vi "Elevator Control Loop.vi"() -> ()   [LabVIEW 2017]
uses:
  <vilib>/Rock Robotics/WPI/MotorControl/WPI_MotorControlDeviceRef.ctl
  <vilib>/Rock Robotics/WPI/MotorControl/WPI_MotorControlType.ctl
  <vilib>/Rock Robotics/SystemInterfaces/DIO/FPGA_DIOPWMChannel.ctl
  <vilib>/Rock Robotics/WPI/PWM/WPI_PWMDeadband.ctl
  <vilib>/Rock Robotics/SystemInterfaces/DIO/FPGA_DIOChannel.ctl
  <vilib>/Rock Robotics/WPI/Encoder/WPI_EncoderDevRef.ctl
  <vilib>/Rock Robotics/SystemInterfaces/Encoder/FPGA_EncoderIdx.ctl
  <vilib>/Rock Robotics/SystemInterfaces/Counter/FPGA_CounterCtrSystemIndex.ctl
  <vilib>/Rock Robotics/WPI/Encoder/WPI_EncoderType.ctl
  Typedef/Controller Message.ctl
  <vilib>/Platform/TimedLoop/XDataNode/timing_clust.ctl
  <vilib>/Platform/TimedLoop/XDataNode/nitl_modes.ctl
  <vilib>/Platform/TimedLoop/XDataNode/wakeup.ctl
  Typedef/FGVAction.ctl
  <vilib>/addons/control/pid/pid.llb/PID Advanced (DBL).vi
  SimulatorVIs/Simulation Input Global.vi
  <vilib>/Platform/TimedLoop/XDataNode/XDataNode.xnode
  <vilib>/Platform/TimedLoop/XDataNode/XDNodeRunTimeDep.lvlib
  <vilib>/addons/control/pid/NI_PID_pid.lvlib
panel:
  in  "min speed":dbl=0.1 format="%#_13g"
  in  "gravity":dbl=0.02 format="%#_13g"
  in  "PIDF gains":cluster{"Kp":dbl, "Ki":dbl, "Kd":dbl, "Kf":dbl}={"Kp"=0.01, "Ki"=0.0, "Kd"=0.06, "Kf"=0.0} {"Kf" format="%.3f"; "Kd" format="%.3f"; "Ki" format="%.3f"; "Kp" format="%.3f"}
  out "Plant Input":dbl(graph)=0.12000000000000001
  in  "output range":cluster{"output high":dbl, "output low":dbl}={"output high"=1.0, "output low"=-1.0} {"output low" format="%.2f"; "output high" format="%.2f"}
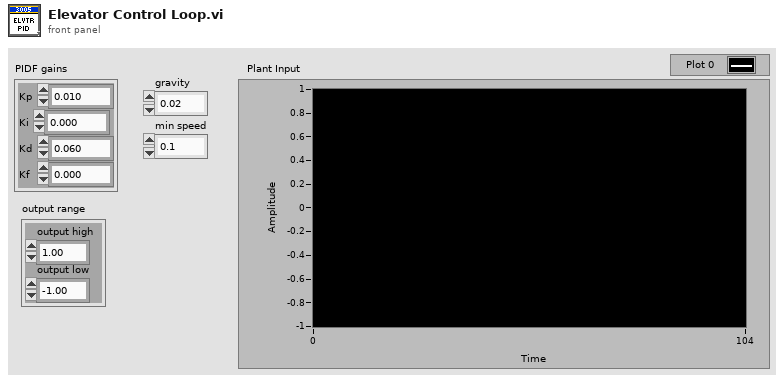
[diagram p1: front panel]
types:
  T1 = typedef "Controller Message.ctl" = cluster{"Setpoint":dbl, "Manual":bool}
  T2 = typedef "WPI_MotorControlDeviceRef.ctl" = cluster{"DeviceStatus":errorcluster, "Type":T3, "PWM":cluster{"PWM Channel":T4, "DeadBand":T5}, "CAN":cluster{"Device Number":u8, "SetOutput VI Ref":variant, "GetOutput VI Ref":variant, "Enable VI Ref":variant, "Disable VI Ref":variant, "Data":variant}, "Invert":bool, "DIO PWM":cluster{"PWM \"Enable\" Channel":T4, "DIOChannel":T6, "PWM Rate":dbl}}
  T3 = typedef "WPI_MotorControlType.ctl" = enum16{"PWM", "CAN", "DIO PWM"}
  T4 = typedef "FPGA_DIOPWMChannel.ctl" = enum8{"PWM 0", "PWM 1", "PWM 2", "PWM 3", "PWM 4", "PWM 5", "PWM 6", "PWM 7", "PWM 8", "PWM 9", "PWM MXP 0", "PWM MXP 1", "PWM MXP 2", "PWM MXP 3", "PWM MXP 4", "PWM MXP 5", "PWM MXP 6", "PWM MXP 7", "PWM MXP 8", "PWM MXP 9", "Invalid"}
  T5 = typedef "WPI_PWMDeadband.ctl" = cluster{"Name":string, "maxPositivePwm":i32, "minPositivePwm":i32, "centerPwm":i32, "maxNegativePwm":i32, "minNegativePwm":i32, "angularRange":u16}
  T6 = typedef "FPGA_DIOChannel.ctl" = enum8{"DIO 0", "DIO 1", "DIO 2", "DIO 3", "DIO 4", "DIO 5", "DIO 6", "DIO 7", "DIO 8", "DIO 9", "DIO MXP 0", "DIO MXP 1", "DIO MXP 2", "DIO MXP 3", "DIO MXP 4", "DIO MXP 5", "DIO MXP 6", "DIO MXP 7", "DIO MXP 8", "DIO MXP 9", "DIO MXP 10", "DIO MXP 11", "DIO MXP 12", "DIO MXP 13", "DIO MXP 14", "DIO MXP 15", "SPI Port CS1", "SPI Port CS2", "SPI Port CS3", "SPI Port MISO", "SPI Port MOSI", "Invalid"}
  T7 = typedef "WPI_EncoderDevRef.ctl" = cluster{"DevStatus":errorcluster, "EncoderIndex":T8, "CounterIndex":T9, "DistancePerCount":dbl, "Decoding Type":T10}
  T8 = typedef "FPGA_EncoderIdx.ctl" = enum8{"Enc 0", "Enc 1", "Enc 2", "Enc 3", "Enc 4", "Enc 5", "Enc 6", "Enc 7", "Invalid"}
  T9 = typedef "FPGA_CounterCtrSystemIndex.ctl" = enum8{"Ctr 0", "Ctr 1", "Ctr 2", "Ctr 3", "Ctr 4", "Ctr 5", "Ctr 6", "Ctr 7", "Invalid"}
  T10 = typedef "WPI_EncoderType.ctl" = enum16{"1x", "2x", "4x"}
  T11 = cluster{"Setpoint":dbl, "Output":dbl, "DriveMotor":T2, "Encoder":T7, "notifier":refnum<notifier>, "Manual?":bool}
  T12 = typedef "XDNodeRunTimeDep.lvlib/timing_clust.ctl" = cluster{"Expected End [f-1]":u64, "Actual End [f-1]":u64, "Finished Late? [f-1]":bool, "Expected End [i-1]":u64, "Actual End [i-1]":u64, "Finished Late? [i-1]":bool, "Expected Start [i]":u64, "Actual Start [i]":u64, "Expected Start [f]":u64, "Actual Start [f]":u64, "Source Name":string, "Structure Name":string, "Period":i64, "Deadline":i64, "Offset":i64, "Start":i64, "Priority":i32, "Timeout":i32, "Mode":T13, "Wakeup Reason":T14, "Error":errorcluster, "Source Type":string, "Secondary Source Type":string, "Global End Time":u64, "Global Start Time":u64, "Frame Duration":u64, "Iteration Duration":u64, "Assigned CPU":i32, "I/O Scan Engine Mode":u32}
  T13 = typedef "XDNodeRunTimeDep.lvlib/nitl_modes.ctl" = enum32{"No Change", "Process missed periods, maintain original phase", "Discard missed periods, maintain original phase", "Process missed periods, ignore original phase", "Discard missed periods, ignore original phase"}
  T14 = typedef "XDNodeRunTimeDep.lvlib/wakeup.ctl" = enum32{"Normal", "Aborted", "Asynchronous wakeup", "Timing source error", "Timed loop error", "Timeout"}
  T15 = typedef "FGVAction.ctl" = enum16{"get", "set"}
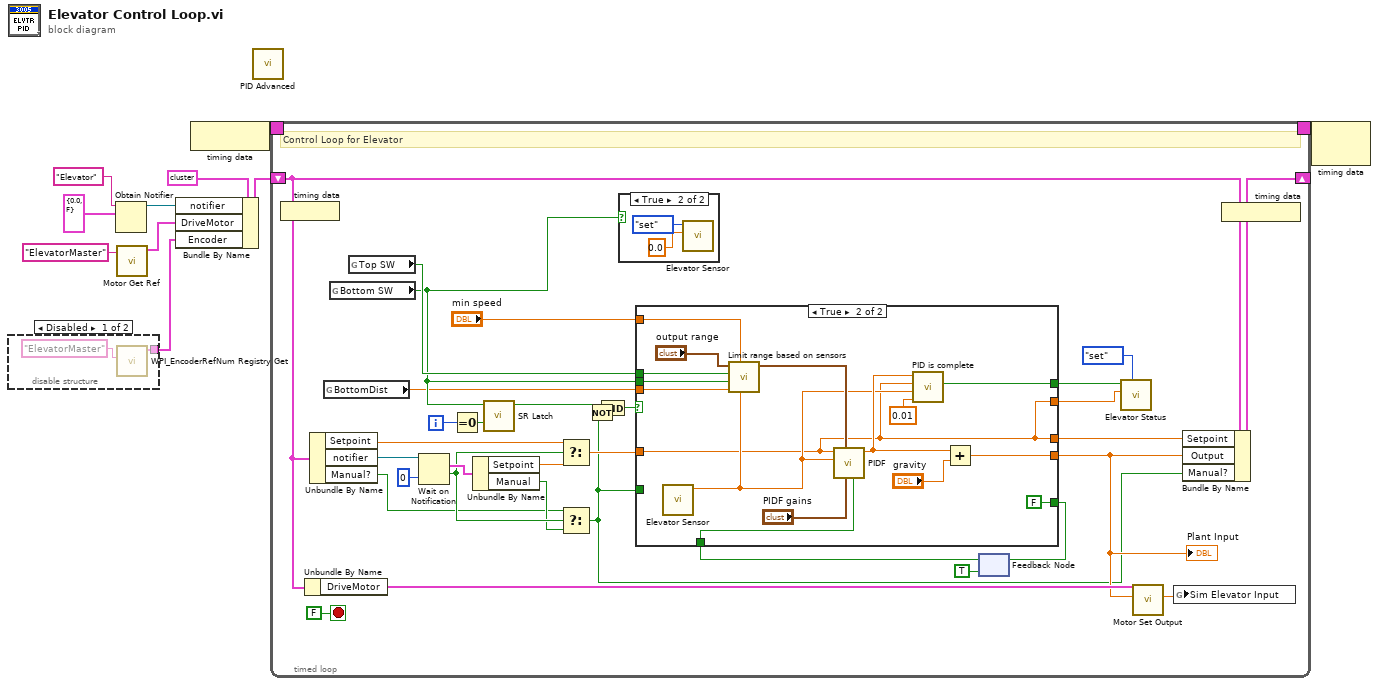
[diagram p0: block diagram]
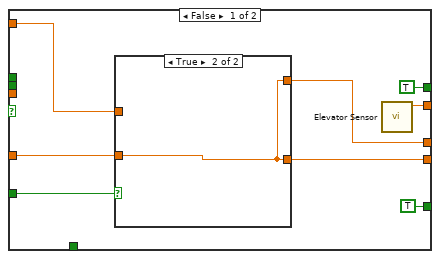
[diagram p3: hidden frame]
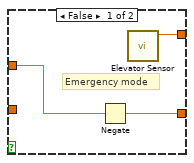
[diagram p4: hidden frame]
diagram:
  n1 = disable-structure shown="Disabled" {
    disable-tunnel: [w11 _] -> w4
    frame Disabled {
      n2 = call <vilib>:"WPI_EncoderRefNum Registry Get.vi"("refnum name"="ElevatorMaster") -> ("EncoderDevRef"=w11:T7)  [unwired: 9 in, 1 out]
    }
    frame Enabled {
    }
  }
  n3 = Obtain Notifier(name (unnamed)="Elevator", notification data type=T1 {"Setpoint"=0.0, "Manual"=FALSE}) -> (notifier out=w8:refnum<notifier>)  [unwired: 2 in, 2 out]
  n4 = call "Motor Get Ref.vi"("refnum name"="ElevatorMaster") -> ("MotorControlDevRef"=w6:T2)  [unwired: 10 in]
  n5 = Bundle By Name(cluster=T11 {"Setpoint"=0.0, "Output"=0.0, "DriveMotor"={"DeviceStatus"={"status"=FALSE, "code"=0, "source"=""}, "Type"=enum."PWM", "PWM"={"PWM Channel"=enum."Invalid", "DeadBand"={"Name"="", "maxPositivePwm"=0, "minPositivePwm"=0, "centerPwm"=0, "maxNegativePwm"=0, "minNegativePwm"=0, "angularRange"=0}}, "CAN"={"Device Number"=0, "SetOutput VI Ref"=variant(enum8{"Percent VBus", "Current", "Speed", "Position", "Voltage"} enum."Percent VBus"), "GetOutput VI Ref"=variant(refnum<k1> refnum), "Enable VI Ref"=variant(dbl 12.0), "Disable VI Ref"=variant(enum8{"Percent VBus", "Speed", "Position", "Slave", "Unchanged / Invalid"} enum."Percent VBus"), "Data"=variant(enum16{"Controller 1"} enum."Controller 1")}, "Invert"=FALSE, "DIO PWM"={"PWM \"Enable\" Channel"=enum."Invalid", "DIOChannel"=enum."Invalid", "PWM Rate"=0.0}}, "Encoder"={"DevStatus"={"status"=FALSE, "code"=0, "source"=""}, "EncoderIndex"=enum."Invalid", "CounterIndex"=enum."Invalid", "DistancePerCount"=1.0, "Decoding Type"=enum."4x"}, "notifier"=refnum, "Manual?"=FALSE}, "notifier"=w8, "DriveMotor"=w6, "Encoder"=w4) -> (w9:T11)
  n6 = node-c288() -> (w3:T12)
  n7 = call-poly <vilib>:"PID Advanced.vi"() -> ()  [unwired: 14 in, 2 out]
  n8 = timed-loop {
    shift-right: [w41] -> _
    shift-left: w9 -> [w18]
    timing: w3 -> [_]
    timing-out: [_] -> w2
    i -> [w31]
    stop <- FALSE stop-if-true
    # "Control Loop for Elevator"
    n9 = node-c288() -> ()  [unwired: 1 in]
    n10 = Unbundle By Name(w18) -> ("DriveMotor"=w39:T2)
    n11 = Unbundle By Name(w18) -> ("Setpoint"=w42:dbl, "notifier"=w43:refnum<notifier>, "Manual?"=w17:bool)
    n12 = global read "Simulation Input Global.vi" "BottomDist"() -> (w32:dbl)
    n13 = global read "Simulation Input Global.vi" "Bottom SW"() -> (w33:bool)
    n14 = global read "Simulation Input Global.vi" "Top SW"() -> (w34:bool)
    n15 = Wait on Notification(notifier=w43, timeout in ms (-1)=0) -> (notification=w22:T1, timed out?=w20:bool)  [unwired: 2 in, 2 out]
    n16 = Equal To 0?(x=w31) -> (x = 0?=w30:bool)
    n17 = Unbundle By Name(w22) -> ("Setpoint"=w21:dbl, "Manual"=w19:bool)
    n18 = call "SR Latch.vi"("Reset"=w30, "Value"=w33) -> ("Latched"=w29:bool)  [unwired: 7 in]
    n19 = Select(t=w42, s=w20, f=w21) -> (s? t:f=w37:dbl)
    n20 = Select(t=w17, s=w20, f=w19) -> (s? t:f=w15:bool)
    n21 = Not(x=w15) -> (.not. x?=w14:bool)
    n22 = And(x=w29, y=w14) -> (x .and. y?=w16:bool)
    n23 = case shown="True" w33 {
      frame False {
      }
      frame True {
        n24 = call "Elevator Sensor.vi"("Value"=0.0, "Action"=FGVAction."set") -> ()  [unwired: 8 in, 2 out]
      }
    }
    n25 = feedback #1(TRUE ("Reinitialize")) -> (w24:bool)
    n26 = case shown="True" w16 {
      tunnel: w37 -> [w47 w57]
      tunnel: "min speed" -> [w52 w68]
      tunnel: [w49 w66] -> w35
      tunnel: w34 -> [_ w64]
      tunnel: w33 -> [_ w63]
      tunnel: w32 -> [_ w62]
      tunnel: [w46 w57] -> w26
      tunnel: [TRUE ("PID is Done?") w60] -> w27
      tunnel: [TRUE ("Reinitialize") FALSE ("Reinitialize?")] -> w25
      tunnel: w24 -> [_ w59]
      tunnel: w15 -> [w48 _]
      tunnel: [w45 w57] -> w13
      frame False {
        n27 = case shown="True" w48 {
          tunnel: w52 -> [w55 _]
          tunnel: [w54 w56] -> w49
          tunnel: w47 -> [_ w56]
          tunnel: [w53 w56] -> w46
          frame False {
            # "Emergency mode"
            n28 = Negate(x=w55) -> (-x=w54:dbl)
            n29 = call "Elevator Sensor.vi"() -> ("Value"=w53:dbl)  [unwired: 10 in, 1 out]
          }
          frame True {
          }
        }
        n30 = call "Elevator Sensor.vi"() -> ("Value"=w45:dbl)  [unwired: 10 in, 1 out]
      }
      frame True {
        n31 = call "Elevator Sensor.vi"() -> ("Value"=w61:dbl)  [unwired: 10 in, 1 out]
        n32 = call "Limit range based on sensors.vi"("Position"=w61, "min speed"=w68, "BottomDist"=w62, "Bottom SW"=w63, "Top SW"=w64, "output range in"="output range") -> ("output range out"=w69:cluster{"output high":dbl, "output low":dbl})  [unwired: 5 in]
        n33 = call "PIDF.vi"("reinitialize? (F)"=w59, "PIDF gains"="PIDF gains", "output range"=w69, "process variable"=w61, "setpoint"=w57) -> ("output"=w71:dbl)  [unwired: 4 in, 2 out]
        n34 = call "PID is complete.vi"("threshold"=0.01, "process variable"=w61, "setpoint"=w57, "PID Output"=w71) -> ("PID is Done?"=w60:bool)  [unwired: 6 in, 1 out]
        n35 = Add(x=w71, y="gravity") -> (x+y=w66:dbl)
      }
    }
    "Plant Input" <- w35
    n36 = feedback-in #1(w25) -> ()
    n37 = call "Elevator Status.vi"("Action"=FGVAction."set", "Input"=w13, "Moving? (F)"=w27) -> ()  [unwired: 6 in, 3 out]
    n38 = call "Motor Set Output.vi"("output"=w35, "DriveMotor"=w39) -> ("Motor Output"=w38:dbl)  [unwired: 9 in]
    n39 = global write "Simulation Input Global.vi" "Sim Elevator Input"(w38) -> ()
    n40 = Bundle By Name(cluster=w18, "Setpoint"=w26, "Output"=w35, "Manual?"=w15) -> (w41:T11)
    n41 = node-c288() -> ()  [unwired: 1 out]
  }
  n42 = node-c288(w2) -> ()  [unwired: 1 out]
